vi "GetSystemChannelValuesForDuration.vi"(8 "error in (no error)":errorcluster, 10 "Duration (s)":dbl, 11 "VeriStandTestCase in":refnum<class "VeriStandTestCase.lvclass">) -> (0 "error out":errorcluster, 2 "System Channel Information List out":T1[](array[typedef]), 3 "VeriStandTestCase out":refnum<class "VeriStandTestCase.lvclass">)   [LabVIEW 2027, in "VeriStandTestCase.lvclass"]
uses:
  VeriStandTestCase.lvclass
  SystemChannelInformation.ctl
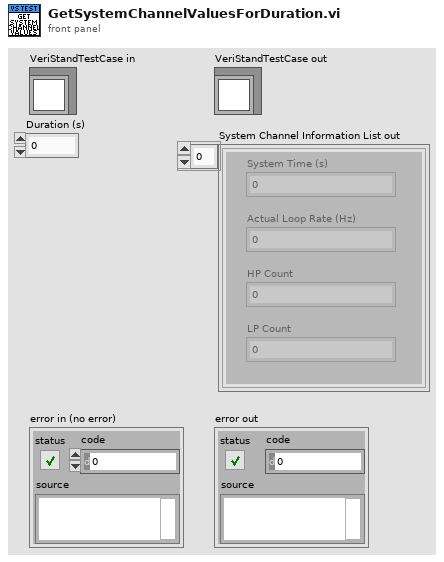
[diagram p1: front panel]
types:
  T1 = typedef "VeriStandTestCase.lvclass/SystemChannelInformation.ctl" = cluster{"Actual Loop Rate (Hz)":dbl, "System Time (s)":dbl, "HP Count":dbl, "LP Count":dbl}
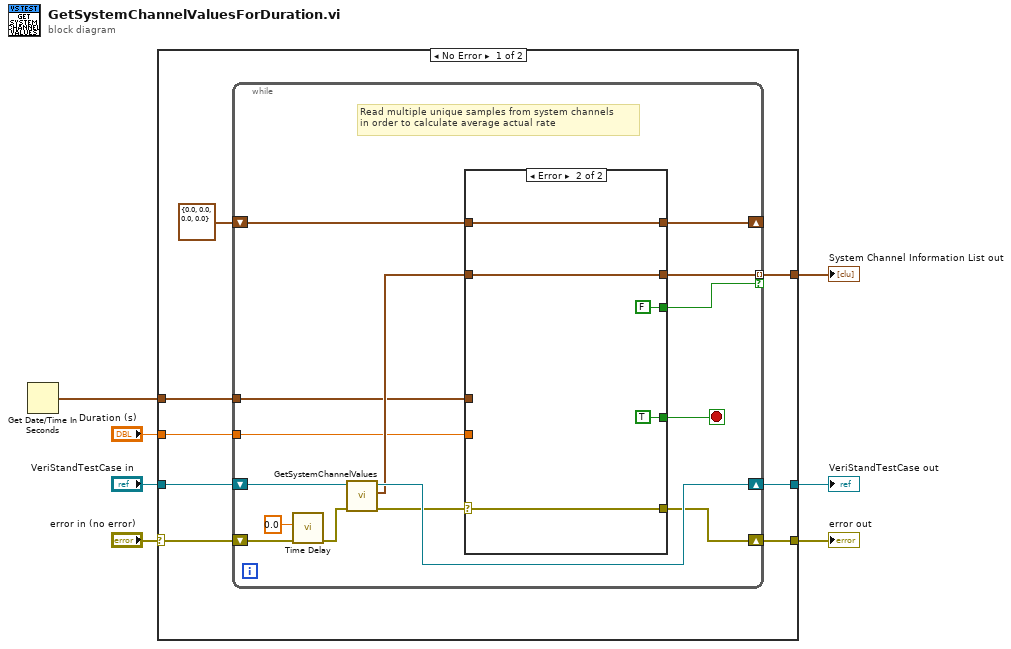
[diagram p0: block diagram]
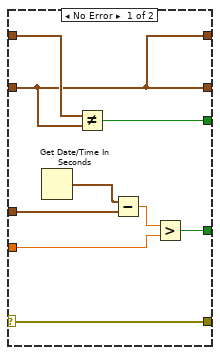
[diagram p2: hidden frame]
diagram:
  n1 = Get Date/Time In Seconds() -> (seconds since 1Jan1904=w3:timestamp)
  n2 = case shown="No Error" "error in (no error)" {
    selector: "error in (no error)" -> [w10 w46]
    tunnel: [w9 _] -> w7
    tunnel: [w15 w45] -> w6
    tunnel: "VeriStandTestCase in" -> [w14 w45]
    tunnel: [w13 w46] -> w4
    tunnel: w3 -> [w12 _]
    tunnel: "Duration (s)" -> [w11 _]
    frame No Error {
      n3 = while {
        shift-right: [w20] -> w13
        shift-left: w10 -> [w28]
        shift-right: [w30] -> w15
        shift-left: w14 -> [w26]
        tunnel: w12 -> [w23]
        tunnel: w11 -> [w22]
        tunnel: [w19] -> w9 mode=indexing if=w17
        shift-right: [w16] -> _
        shift-left: T1 {"Actual Loop Rate (Hz)"=0.0, "System Time (s)"=0.0, "HP Count"=0.0, "LP Count"=0.0} ("System Channel Information") -> [w18]
        stop <- w21 stop-if-true
        # "Read multiple unique samples from system channels\nin order to calculate average actual rate"
        n4 = call "Time Delay"("error in (no error)"=w28, "Delay Time (s)"=0.0) -> ("error out"=w27:errorcluster)  [unwired: 9 in]
        n5 = call "GetSystemChannelValues.vi"("error in (no error)"=w27, "VeriStandTestCase in"=w26) -> ("error out"=w24:errorcluster, "System Channel Information"=w29:T1, "VeriStandTestCase out"=w30:refnum<class "VeriStandTestCase.lvclass">)  [unwired: 7 in]
        n6 = case shown="Error" w24 {
          selector: w24 -> [w34 w43]
          tunnel: w29 -> [w31 w42]
          tunnel: w23 -> [w38 _]
          tunnel: w22 -> [w36 _]
          tunnel: [w35 TRUE] -> w21
          tunnel: [w34 w43] -> w20
          tunnel: [w31 w42] -> w19
          tunnel: w18 -> [w32 w40]
          tunnel: [w33 FALSE] -> w17
          tunnel: [w31 w40] -> w16
          frame No Error {
            n7 = Get Date/Time In Seconds() -> (seconds since 1Jan1904=w39:timestamp)
            n8 = Not Equal?(x=w32, y=w31) -> (x != y?=w33:bool)
            n9 = Subtract(x=w39, y=w38) -> (x-y=w37:dbl)
            n10 = Greater?(x=w37, y=w36) -> (0:w35:bool)
          }
          frame Error {
          }
        }
      }
    }
    frame Error {
    }
  }
  "System Channel Information List out" <- w7
  "VeriStandTestCase out" <- w6
  "error out" <- w4
